vi "4_Factorial(170382,170307).vi"() -> ()   [LabVIEW 2015]
panel:
  in  "Numeric":i64
  out "Numeric 2":u64
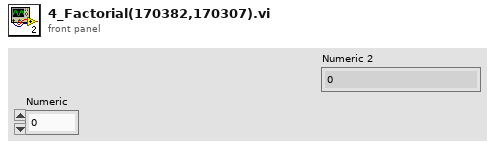
[diagram p1: front panel]
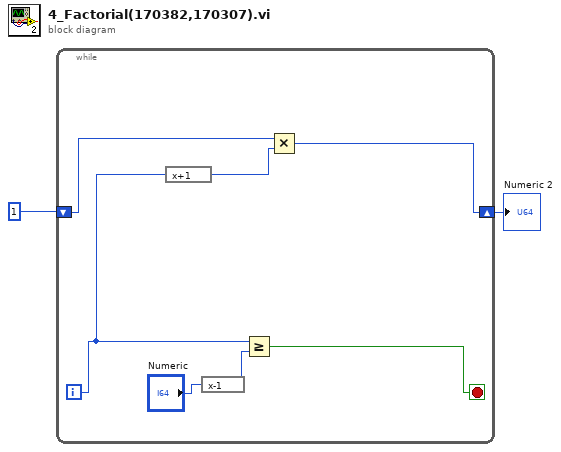
[diagram p0: block diagram]
diagram:
  n1 = while {
    shift-right: [w7] -> w1
    shift-left: u64 1 -> [w8]
    i -> [w5]
    stop <- w9 stop-if-true
    n2 = expression code="x+1"(w5) -> (w6:i32)
    n3 = expression code="x-1"("Numeric") -> (w3:i64)
    n4 = Greater Or Equal?(x=w5, y=w3) -> (x >= y?=w9:bool)
    n5 = Multiply(x=w8, y=w6) -> (x*y=w7:u64)
  }
  "Numeric 2" <- w1
